vi "Update HWplugin List.vi"(8 "error in (no error)":errorcluster, 10 "Array of HWtype\\HWplugin":string[](array[string]), 11 "Operator UI in":refnum<class "Controller UI.lvclass">) -> (0 "error out":errorcluster, 3 "Operator UI out":refnum<class "Controller UI.lvclass">)   [LabVIEW 2016, in "Controller UI.lvlib" / "Controller UI.lvclass"]
uses:
  <userlib>/Common Components/Controller UI/Controller UI.lvclass
  <userlib>/Common Components/Controller UI/Update DT event data.ctl
  <userlib>/Common Components/Controller UI/Update DT Cmd.ctl
  <userlib>/Common Components/Controller UI/Controller UI.lvclass/Controller UI.ctl
  <userlib>/Common Components/Controller UI/Accessors/Write Array of HWtype_HWplugin.vi
  <userlib>/Common Components/Controller UI/Accessors/Read Update DT event.vi
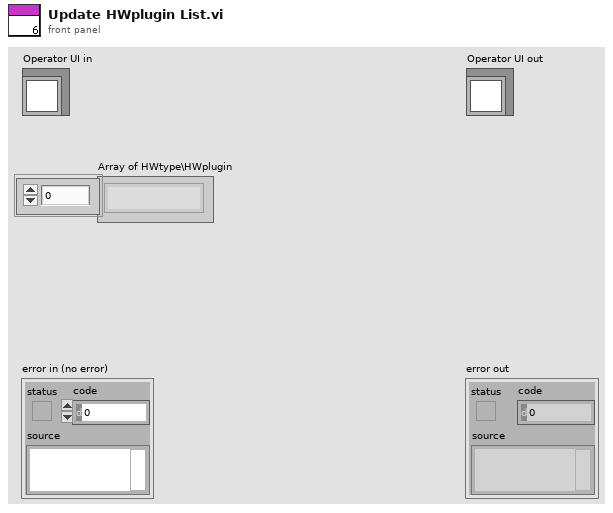
[diagram p1: front panel]
types:
  T1 = typedef "Controller UI.lvlib/Controller UI.lvclass/Update DT event data.ctl" = cluster{"Cmd":T2, "Data Array":variant[]}
  T2 = typedef "Controller UI.lvlib/Controller UI.lvclass/Update DT Cmd.ctl" = enum16{"Update HWtype\\HWplugin array", "Update Checked-out", "Update COMM Status"}
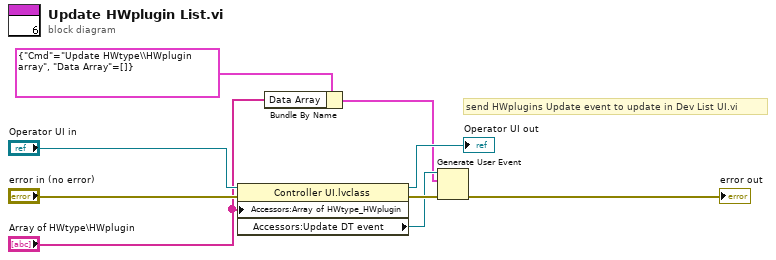
[diagram p0: block diagram]
diagram:
  # "send HWplugins Update event to update in Dev List UI.vi"
  n1 = property class="Controller UI.lvclass"(reference="Operator UI in", error in="error in (no error)", "Accessors:Array of HWtype_HWplugin"="Array of HWtype\\HWplugin") -> (reference out=→"Operator UI out":refnum<class "Controller UI.lvclass">, error out=w7:errorcluster, "Accessors:Update DT event"=w4:refnum<user-event>)
  n2 = Bundle By Name(cluster=T1 {"Cmd"=enum."Update HWtype\\HWplugin array", "Data Array"=[]} ("event data"), "Data Array"="Array of HWtype\\HWplugin") -> (w2:T1)
  n3 = Generate User Event(user event=w4, event data cluster=w2, error in=w7) -> (error out=→"error out":errorcluster)  [unwired: 1 in, 1 out]
